vi "Scope_V1_0.vi"() -> ()   [LabVIEW 2011]
uses:
  GlobalVariable/strGlobalVariable.vi
panel:
  out "strResultArrayOut_1st":string[](array[string])
  out "Chart":T1(graph)
  out "strArrayOut":string[](array[string])
  out "mu32ArrayOut":u32[](array[numeric])
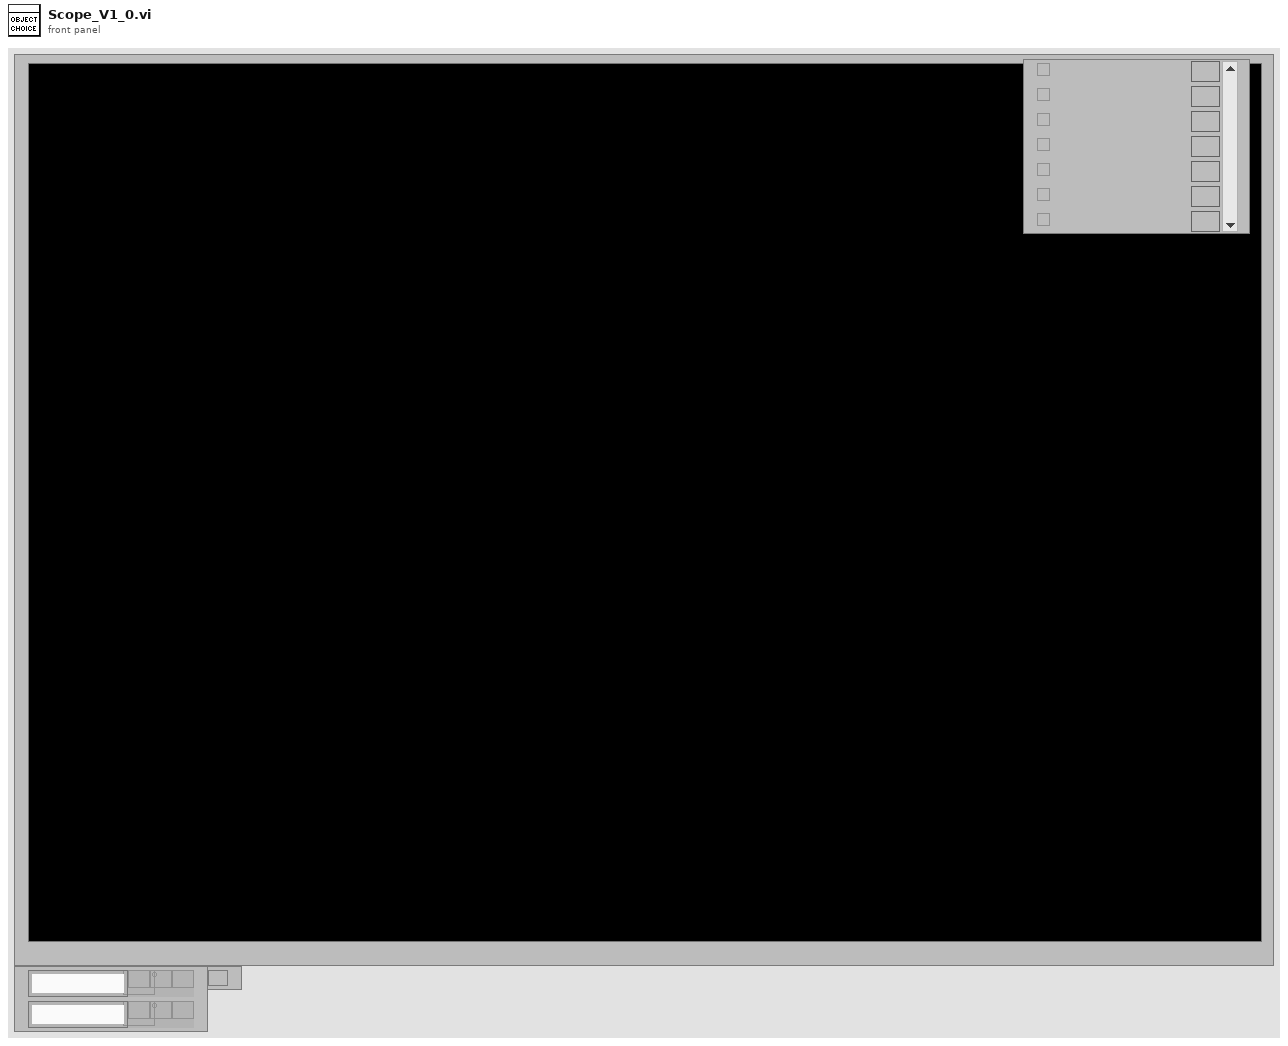
[diagram p1: front panel]
types:
  T1 = cluster{"Value[0]":u32, "Value[1]":u32, "Value[2]":u32, "Value[3]":u32, "Value[4]":u32, "Value[5]":u32, "Value[6]":u32, "Value[7]":u32, "Value[8]":u32, "Value[9]":u32, "Value[10]":u32, "Value[11]":u32, "Value[12]":u32, "Value[13]":u32, "Value[14]":u32, "Value[15]":u32, "Value[16]":u32, "Value[17]":u32, "Value[18]":u32, "Value[19]":u32, "Value[20]":u32, "Value[21]":u32, "Value[22]":u32, "Value[23]":u32, "Value[24]":u32, "Value[25]":u32, "Value[26]":u32, "Value[27]":u32, "Value[28]":u32, "Value[29]":u32, "Value[30]":u32, "Value[31]":u32, "Value[32]":u32, "Value[33]":u32, "Value[34]":u32, "Value[35]":u32, "Value[36]":u32, "Value[37]":u32, "Value[38]":u32, "Value[39]":u32, "Value[40]":u32, "Value[41]":u32, "Value[42]":u32, "Value[43]":u32, "Value[44]":u32, "Value[45]":u32, "Value[46]":u32, "Value[47]":u32, "Value[48]":u32, "Value[49]":u32, "Value[50]":u32, "Value[51]":u32, "Value[52]":u32, "Value[53]":u32, "Value[54]":u32, "Value[55]":u32, "Value[56]":u32, "Value[57]":u32, "Value[58]":u32, "Value[59]":u32, "Value[60]":u32, "Value[61]":u32, "Value[62]":u32, "Value[63]":u32, "Value[64]":u32, "Value[65]":u32, "Value[66]":u32, "Value[67]":u32, "Value[68]":u32, "Value[69]":u32, "Value[70]":u32, "Value[71]":u32, "Value[72]":u32, "Value[73]":u32, "Value[74]":u32, "Value[75]":u32, "Value[76]":u32, "Value[77]":u32, "Value[78]":u32, "Value[79]":u32, "Value[80]":u32}
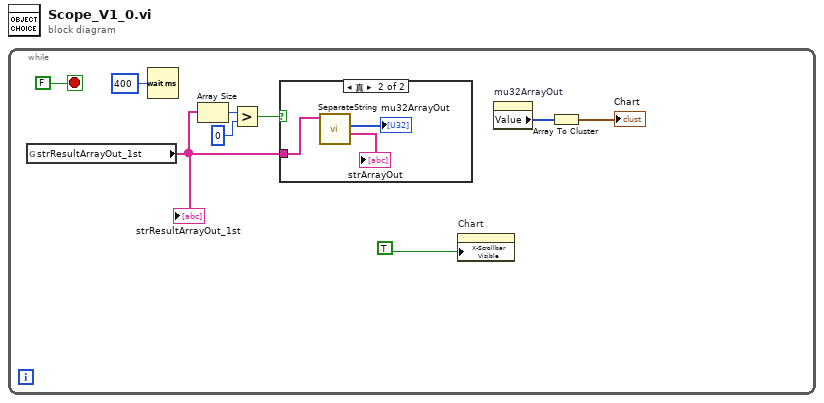
[diagram p0: block diagram]
diagram:
  n1 = while {
    stop <- FALSE stop-if-true
    n2 = global read "strGlobalVariable.vi" "strResultArrayOut_1st"() -> (w3:string[])
    "strResultArrayOut_1st" <- w3
    n3 = Wait (ms)(milliseconds to wait=u32 400 ("等待时间（毫秒）")) -> ()  [unwired: 1 out]
    n4 = Array Size(array=w3) -> (size(s)=w8:i32)
    n5 = Greater?(x=w8, y=0) -> (0:w6:bool)
    n6 = case shown="真" w6 {
      tunnel: w3 -> [_ w12]
      frame False {
      }
      frame True {
        n7 = call "SeparateString.vi"("strArrayIn"=w12) -> ("strArrayOut"=→"strArrayOut":string[], "mu32ArrayOut"=→"mu32ArrayOut":u32[])  [unwired: 8 in, 1 out]
      }
    }
    n8 = property on="Chart" class="WFChart (严格)"("X-Scrollbar Visible"=TRUE ("X滚动条可见")) -> ()  [unwired: 2 in, 2 out]
    n9 = property on="mu32ArrayOut" class="Arr (严格)"() -> ("Value"=w1:u32[])  [unwired: 2 in, 2 out]
    n10 = Array To Cluster(array=w1) -> (cluster=→"Chart":T1)
  }
